vi "GestureRecognition.vi"() -> (3 "KinectOutput":T1)   [LabVIEW 2011]
uses:
  <vilib>/addons/Kinect/Skeleton Vertex Index.ctl
  KinectInputs.ctl
panel:
  out "BothHandsForward":bool=TRUE
  out "RightElbowYZ":dbl
  out "LeftElbowYZ":dbl
  out "AngleArmpitRight":dbl
  out "AngleArmpitLeft":dbl
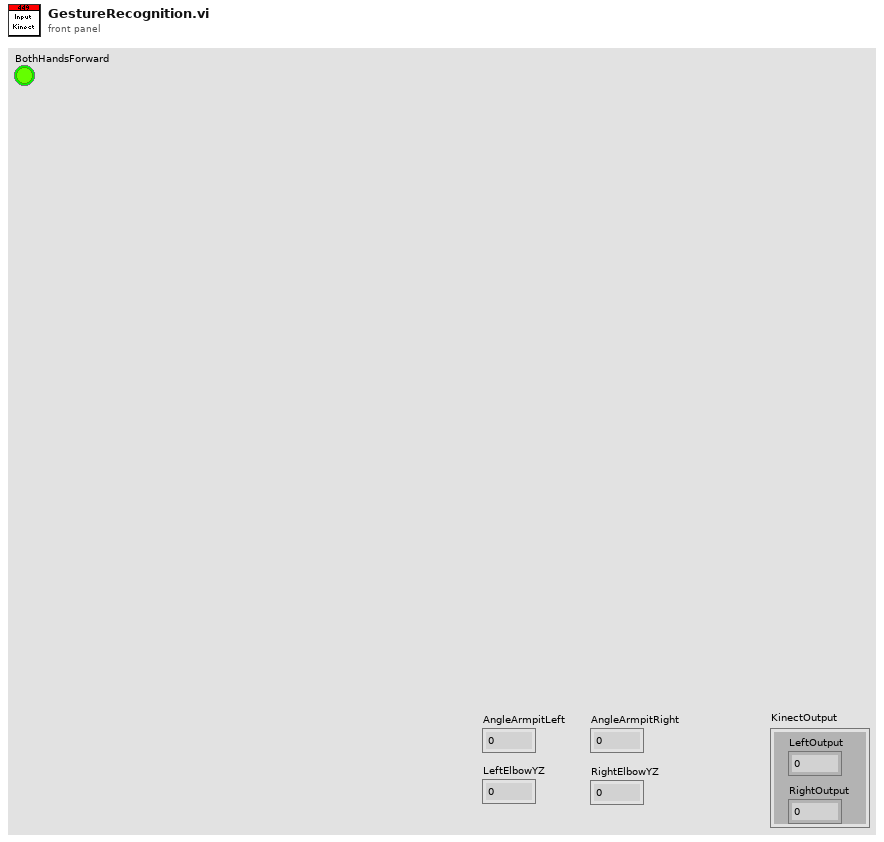
[diagram p1: front panel]
types:
  T1 = typedef "KinectInputs.ctl" = cluster{"LeftOutput":dbl, "RightOutput":dbl}
  T2 = typedef "Skeleton Vertex Index.ctl" = i32
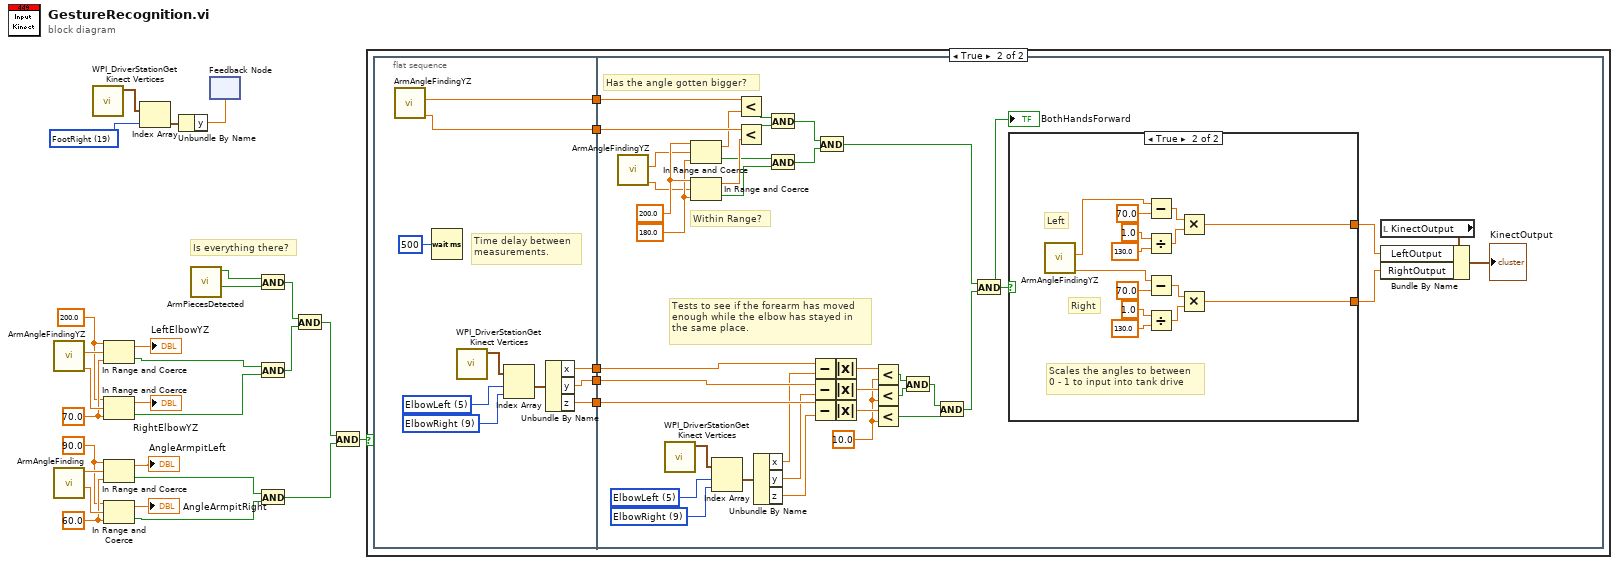
[diagram p0: block diagram]
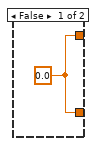
[diagram p3: hidden frame]
diagram:
  w3 = T2 19 items=["HipCenter", "Spine", "ShoulderCenter", "Head", "ShoulderLeft", "ElbowLeft", "WristLeft", "HandLeft", "ShoulderRight", "ElbowRight", "WristRight", "HandRight", "HipLeft", "KneeLeft", "AnkleLeft", "FootLeft", "HipRight", "KneeRight", "AnkleRight", "FootRight"] ("Skeleton Joints")
  w9 = 200.0 ("x")
  w10 = 70.0 ("y")
  w5 = 90.0 ("y")
  w6 = 60.0 ("y")
  # "Is everything there?"
  n1 = call "ArmAngleFindingYZ.vi"() -> ("AngleElbowRight"=w11:dbl, "AngleElbowLeft"=w12:dbl)  [unwired: 7 in, 2 out]
  n2 = call "ArmAngleFinding.vi"() -> ("AngleArmpitRight"=w7:dbl, "AngleArmpitLeft"=w8:dbl)  [unwired: 7 in, 2 out]
  n3 = call <vilib>:"WPI_DriverStationGet Kinect Vertices.vi"() -> ("Skeleton Vertices"=w4:cluster{"x":sgl, "y":sgl, "z":sgl}[])  [unwired: 10 in, 1 out]
  n4 = In Range and Coerce(upper limit=w9, x=w12, lower limit=w10) -> (coerced(x)=→"LeftElbowYZ":dbl, In Range?=w19:bool)
  n5 = In Range and Coerce(upper limit=w9, x=w11, lower limit=w10) -> (coerced(x)=→"RightElbowYZ":dbl, In Range?=w20:bool)
  n6 = In Range and Coerce(upper limit=w5, x=w8, lower limit=w6) -> (coerced(x)=→"AngleArmpitLeft":dbl, In Range?=w15:bool)
  n7 = In Range and Coerce(upper limit=w5, x=w7, lower limit=w6) -> (coerced(x)=→"AngleArmpitRight":dbl, In Range?=w16:bool)
  n8 = Index Array(array=w4, index=w3) -> (element=w2:cluster{"x":sgl, "y":sgl, "z":sgl})
  n9 = Unbundle By Name(w2) -> ("y"=w1:sgl)
  n10 = call "ArmPiecesDetected.vi"() -> ("LeftTracked?"=w21:bool, "RightTracked?"=w22:bool)  [unwired: 10 in]
  n11 = feedback-in #1() -> ()  [unwired: 1 out]
  n12 = feedback #1(w1) -> ()  [unwired: 1 in]
  n13 = And(x=w22, y=w21) -> (x .and. y?=w24:bool)
  n14 = And(x=w19, y=w20) -> (x .and. y?=w23:bool)
  n15 = And(x=w15, y=w16) -> (x .and. y?=w26:bool)
  n16 = And(x=w24, y=w23) -> (x .and. y?=w25:bool)
  n17 = And(x=w25, y=w26) -> (x .and. y?=w27:bool)
  n18 = case shown="True" w27 {
    frame False {
    }
    frame True {
      n19 = flat-sequence {
        tunnel: [w41] -> w32
        tunnel: [w40] -> w31
        tunnel: [w35] -> w30
        tunnel: [w34] -> w29
        tunnel: [w33] -> w28
        tunnel: w32 -> [w80]
        tunnel: w31 -> [w79]
        tunnel: w30 -> [w66]
        tunnel: w29 -> [w65]
        tunnel: w28 -> [w64]
        frame #0 {
          w36 = T2 9 items=["HipCenter", "Spine", "ShoulderCenter", "Head", "ShoulderLeft", "ElbowLeft", "WristLeft", "HandLeft", "ShoulderRight", "ElbowRight", "WristRight", "HandRight", "HipLeft", "KneeLeft", "AnkleLeft", "FootLeft", "HipRight", "KneeRight", "AnkleRight", "FootRight"] ("Skeleton Joints")
          w39 = T2 5 items=["HipCenter", "Spine", "ShoulderCenter", "Head", "ShoulderLeft", "ElbowLeft", "WristLeft", "HandLeft", "ShoulderRight", "ElbowRight", "WristRight", "HandRight", "HipLeft", "KneeLeft", "AnkleLeft", "FootLeft", "HipRight", "KneeRight", "AnkleRight", "FootRight"] ("Skeleton Joints")
          # "Time delay between\nmeasurements."
          n20 = call "ArmAngleFindingYZ.vi"() -> ("AngleElbowRight"=w40:dbl, "AngleElbowLeft"=w41:dbl)  [unwired: 7 in, 2 out]
          n21 = Wait (ms)(milliseconds to wait=u32 500) -> ()  [unwired: 1 out]
          n22 = call <vilib>:"WPI_DriverStationGet Kinect Vertices.vi"() -> ("Skeleton Vertices"=w38:cluster{"x":sgl, "y":sgl, "z":sgl}[])  [unwired: 10 in, 1 out]
          n23 = Index Array(array=w38, index #1=w39, index #2=w36) -> (element #1=w37:cluster{"x":sgl, "y":sgl, "z":sgl})  [unwired: 1 out]
          n24 = Unbundle By Name(w37) -> ("x"=w35:sgl, "y"=w34:sgl, "z"=w33:sgl)
        }
        frame #1 {
          w57 = sgl 10.0 ("y")
          w71 = T2 9 items=["HipCenter", "Spine", "ShoulderCenter", "Head", "ShoulderLeft", "ElbowLeft", "WristLeft", "HandLeft", "ShoulderRight", "ElbowRight", "WristRight", "HandRight", "HipLeft", "KneeLeft", "AnkleLeft", "FootLeft", "HipRight", "KneeRight", "AnkleRight", "FootRight"] ("Skeleton Joints")
          w74 = T2 5 items=["HipCenter", "Spine", "ShoulderCenter", "Head", "ShoulderLeft", "ElbowLeft", "WristLeft", "HandLeft", "ShoulderRight", "ElbowRight", "WristRight", "HandRight", "HipLeft", "KneeLeft", "AnkleLeft", "FootLeft", "HipRight", "KneeRight", "AnkleRight", "FootRight"] ("Skeleton Joints")
          w83 = 180.0 ("x")
          w84 = 200.0 ("x")
          # "Has the angle gotten bigger?"
          # "Within Range?"
          # "Tests to see if the forearm has moved\nenough while the elbow has stayed in\nthe same place."
          n25 = call "ArmAngleFindingYZ.vi"() -> ("AngleElbowRight"=w82:dbl, "AngleElbowLeft"=w81:dbl)  [unwired: 7 in, 2 out]
          n26 = call <vilib>:"WPI_DriverStationGet Kinect Vertices.vi"() -> ("Skeleton Vertices"=w73:cluster{"x":sgl, "y":sgl, "z":sgl}[])  [unwired: 10 in, 1 out]
          n27 = In Range and Coerce(upper limit=w84, x=w81, lower limit=w83) -> (coerced(x)=w76:dbl, In Range?=w52:bool)
          n28 = In Range and Coerce(upper limit=w84, x=w82, lower limit=w83) -> (coerced(x)=w75:dbl, In Range?=w70:bool)
          n29 = Index Array(array=w73, index #1=w74, index #2=w71) -> (element #1=w72:cluster{"x":sgl, "y":sgl, "z":sgl})  [unwired: 1 out]
          n30 = Less?(x=w80, y=w76) -> (x < y?=w77:bool)
          n31 = Less?(x=w79, y=w75) -> (x < y?=w78:bool)
          n32 = Unbundle By Name(w72) -> ("x"=w63:sgl, "y"=w61:sgl, "z"=w62:sgl)
          n33 = And(x=w77, y=w78) -> (x .and. y?=w49:bool)
          n34 = And(x=w52, y=w70) -> (x .and. y?=w48:bool)
          n35 = Subtract(x=w66, y=w63) -> (x-y=w69:sgl)
          n36 = Subtract(x=w65, y=w61) -> (x-y=w68:sgl)
          n37 = Subtract(x=w64, y=w62) -> (x-y=w67:sgl)
          n38 = And(x=w49, y=w48) -> (x .and. y?=w50:bool)
          n39 = Absolute Value(x=w69) -> (abs(x)=w60:sgl)
          n40 = Absolute Value(x=w68) -> (abs(x)=w59:sgl)
          n41 = Absolute Value(x=w67) -> (abs(x)=w58:sgl)
          n42 = Less?(x=w60, y=w57) -> (x < y?=w55:bool)
          n43 = Less?(x=w59, y=w57) -> (x < y?=w56:bool)
          n44 = Less?(x=w58, y=w57) -> (x < y?=w53:bool)
          n45 = And(x=w55, y=w56) -> (x .and. y?=w54:bool)
          n46 = And(x=w54, y=w53) -> (x .and. y?=w51:bool)
          n47 = And(x=w50, y=w51) -> (x .and. y?=w43:bool)
          "BothHandsForward" <- w43
          n48 = case shown="True" w43 {
            tunnel: [w85 w87] -> w45
            tunnel: [w85 w86] -> w44
            frame False {
              w85 = 0.0
            }
            frame True {
              # "Left"
              # "Right"
              # "Scales the angles to between \n0 - 1 to input into tank drive"
              n49 = call "ArmAngleFindingYZ.vi"() -> ("AngleElbowRight"=w89:dbl, "AngleElbowLeft"=w88:dbl)  [unwired: 7 in, 2 out]
              n50 = Subtract(x=w88, y=70.0) -> (x-y=w91:dbl)
              n51 = Divide(x=1.0, y=130.0) -> (x/y=w90:dbl)
              n52 = Subtract(x=w89, y=70.0) -> (x-y=w96:dbl)
              n53 = Divide(x=1.0, y=130.0) -> (x/y=w95:dbl)
              n54 = Multiply(x=w91, y=w90) -> (x*y=w87:dbl)
              n55 = Multiply(x=w96, y=w95) -> (x*y=w86:dbl)
            }
          }
          n56 = local read "KinectOutput"() -> (w46:T1)
          n57 = Bundle By Name(cluster=w46, "LeftOutput"=w45, "RightOutput"=w44) -> (→"KinectOutput":T1)
        }
      }
    }
  }
